vi "Lambda_Configuration4.vi"() -> ()   [LabVIEW 2015]
uses:
  <vilib>/Utility/error.llb/DialogType.ctl
  <vilib>/Platform/TimedLoop/XDataNode/timing_clust.ctl
  <vilib>/Platform/TimedLoop/XDataNode/nitl_modes.ctl
  <vilib>/Platform/TimedLoop/XDataNode/wakeup.ctl
  <vilib>/Utility/file.llb/Read From Spreadsheet File (DBL).vi
  <vilib>/platform/TimedLoop/XDataNode/XDataNode.xnode
  <vilib>/Platform/TimedLoop/XDataNode/XDNodeRunTimeDep.lvlib
panel:
  in  "?":bool
  out "Voltage":dbl[](graph)
  out "Current":dbl[](graph)
  in  "?":bool
  out "Output Current":dbl format="%.4f"
  out "Output Voltage":dbl format="%.4f"
  out "Serial Number:":string
  out "error?":bool
  out "Model:":string
  in  "Reset (T)":bool=TRUE
  in  "BAUD":u16(ring)=3 items=["1200", "2400", "4800", "9600", "19200"]
  in  "GEN Addr":i16=6
  in  "VISA name":refnum<visa-resource-name>
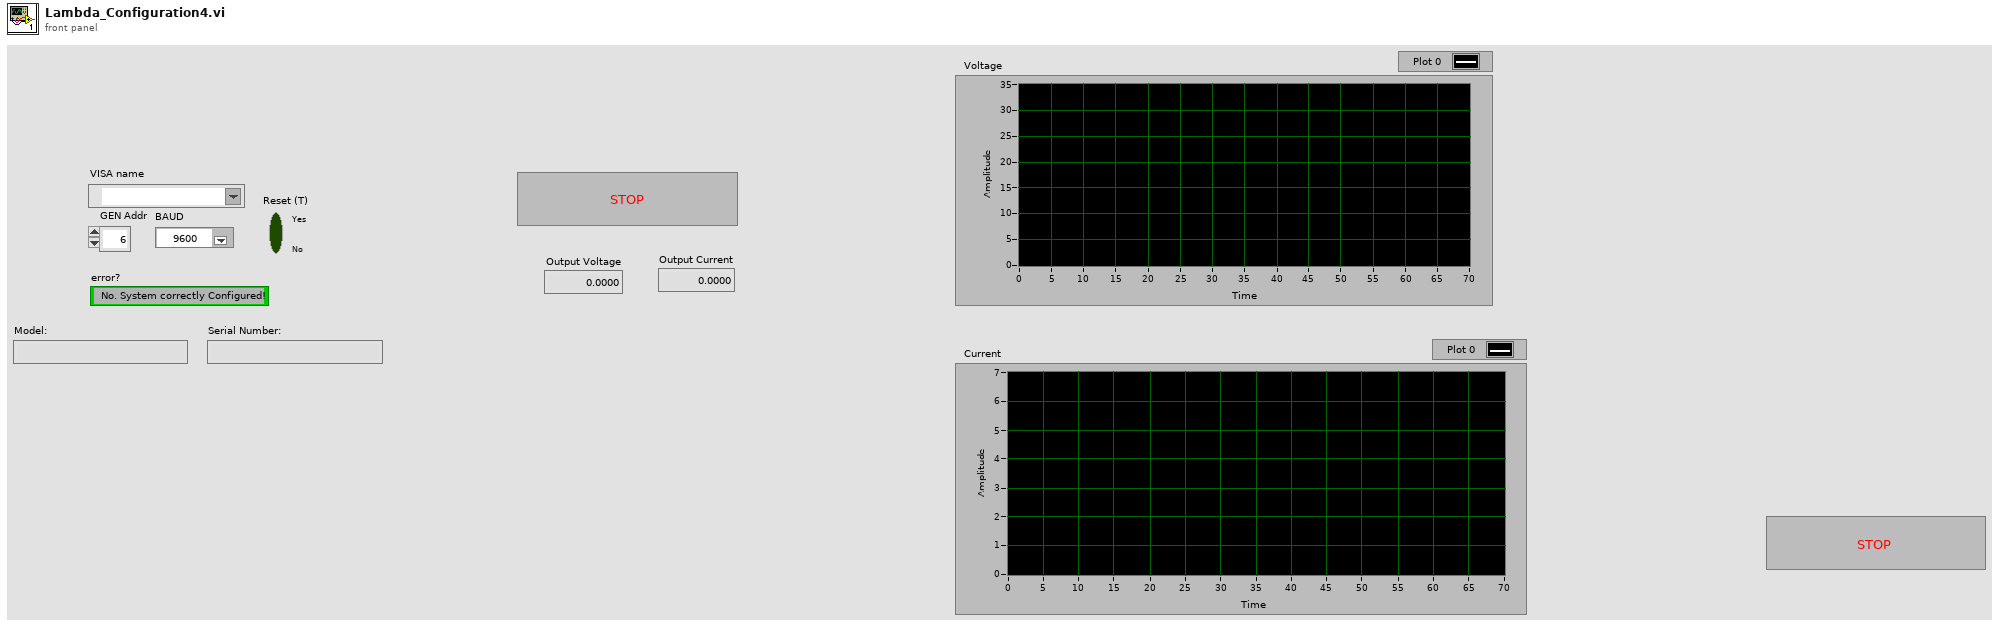
[diagram p1: front panel]
types:
  T1 = typedef "XDNodeRunTimeDep.lvlib/timing_clust.ctl" = cluster{"Expected End [f-1]":u64, "Actual End [f-1]":u64, "Finished Late? [f-1]":bool, "Expected End [i-1]":u64, "Actual End [i-1]":u64, "Finished Late? [i-1]":bool, "Expected Start [i]":u64, "Actual Start [i]":u64, "Expected Start [f]":u64, "Actual Start [f]":u64, "Source Name":string, "Structure Name":string, "Period":i64, "Deadline":i64, "Offset":i64, "Start":i64, "Priority":i32, "Timeout":i32, "Mode":T2, "Wakeup Reason":T3, "Error":errorcluster, "Source Type":string, "Secondary Source Type":string, "Global End Time":u64, "Global Start Time":u64, "Frame Duration":u64, "Iteration Duration":u64, "Assigned CPU":i32, "I/O Scan Engine Mode":u32}
  T2 = typedef "XDNodeRunTimeDep.lvlib/nitl_modes.ctl" = enum32{"No Change", "Process missed periods, maintain original phase", "Discard missed periods, maintain original phase", "Process missed periods, ignore original phase", "Discard missed periods, ignore original phase"}
  T3 = typedef "XDNodeRunTimeDep.lvlib/wakeup.ctl" = enum32{"Normal", "Aborted", "Asynchronous wakeup", "Timing source error", "Timed loop error", "Timeout"}
  T4 = typedef "DialogType.ctl" = u16
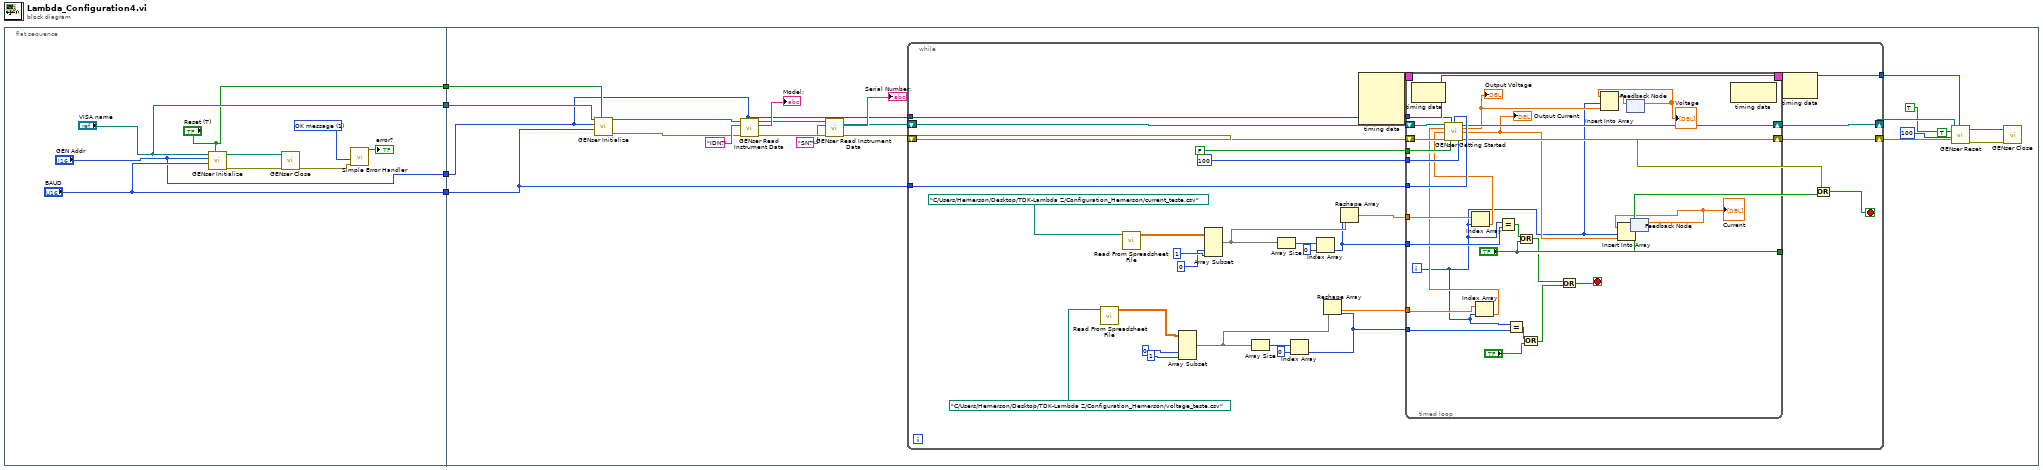
[diagram p0: block diagram]
diagram:
  n1 = flat-sequence {
    tunnel: ["BAUD"] -> w4
    tunnel: ["GEN Addr"] -> w3
    tunnel: ["VISA name"] -> w2
    tunnel: ["Reset (T)"] -> w1
    tunnel: w4 -> [w21]
    tunnel: w3 -> [w22]
    tunnel: w2 -> [w27]
    tunnel: w1 -> [w28]
    frame #0 {
      w10 = T4 1 items=["no dialog", "OK message", "continue or stop message", "OK message + warnings", "continue/stop + warnings"] ("type of dialog (OK msg:1)")
      n2 = call <instrlib>:"GENser Initialize.vi"("Reset (T)"="Reset (T)", "BAUD"="BAUD", "GEN Addr"="GEN Addr", "VISA name"="VISA name") -> ("error out"=w12:errorcluster, "VISA out"=w13:refnum<visa-resource-name>)  [unwired: 6 in]
      n3 = call <instrlib>:"GENser Close.vi"("error"=w12, "VISA name"=w13) -> ("error out"=w11:errorcluster)  [unwired: 9 in]
      n4 = call <vilib>:"Simple Error Handler.vi"("type of dialog (OK msg:1)"=w10, "error in (no error)"=w11) -> ("error?"=→"error?":bool)  [unwired: 3 in, 4 out]
    }
    frame #1 {
      (unwired) TRUE ("Reset (T)")
      n5 = call <instrlib>:"GENser Initialize.vi"("Reset (T)"=w28, "BAUD"=w21, "GEN Addr"=w22, "VISA name"=w27) -> ("error out"=w25:errorcluster, "VISA out"=w26:refnum<visa-resource-name>)  [unwired: 6 in]
      n6 = call <instrlib>:"GENser Read Instrument Data.vi"("GEN Addr"=w22, "error"=w25, "Query"="IDN?", "VISA"=w26) -> ("error out"=w31:errorcluster, "Response"=→"Model:":string, "VISA out"=w32:refnum<visa-resource-name>)  [unwired: 4 in, 1 out]
      n7 = call <instrlib>:"GENser Read Instrument Data.vi"("error"=w31, "Query"="SN?", "VISA"=w32) -> ("error out"=w23:errorcluster, "Response"=→"Serial Number:":string, "VISA out"=w24:refnum<visa-resource-name>)  [unwired: 5 in, 1 out]
      n8 = while {
        tunnel: w22 -> [w57]
        tunnel: w21 -> [w61]
        shift-right: [w58] -> w20
        shift-left: w24 -> [w64]
        shift-right: [w47] -> w19
        shift-left: w23 -> [w62]
        tunnel: [w57] -> w16
        stop <- w60 stop-if-true
        n9 = call-poly <vilib>:"Read From Spreadsheet File.vi"("file path (dialog if empty)"=path "C:/Users/Hemerson/Desktop/TDK-Lambda Z/Configuration_Hemerson/voltage_teste.csv") -> ("all rows"=w35:dbl[][])  [unwired: 6 in, 4 out]
        n10 = call-poly <vilib>:"Read From Spreadsheet File.vi"("file path (dialog if empty)"=path "C:/Users/Hemerson/Desktop/TDK-Lambda Z/Configuration_Hemerson/current_teste.csv") -> ("all rows"=w42:dbl[][])  [unwired: 6 in, 4 out]
        n11 = Array Subset "Array Subset"(array=w35, index (col)=0 ("index"), length (col)=1 ("length")) -> (w39:dbl[][])  [unwired: 2 in]
        n12 = Array Subset "Array Subset"(array=w42, index (col)=0 ("index"), length (col)=1 ("length")) -> (w53:dbl[][])  [unwired: 2 in]
        n13 = Array Size(array=w39) -> (size(s)=w43:i32[])
        n14 = Array Size(array=w53) -> (size(s)=w54:i32[])
        n15 = Index Array "Index Array"(array=w43, index=0) -> (element=w38:i32)
        n16 = Index Array "Index Array"(array=w54, index=0) -> (element=w46:i32)
        n17 = Reshape Array "Reshape Array"(w39, w38) -> (w37:dbl[])
        n18 = Reshape Array "Reshape Array"(w53, w46) -> (w48:dbl[])
        n19 = node-c288() -> (w50:T1)  [unwired: 4 in]
        n20 = timed-loop {
          timing: w50 -> [_]
          timing-out: [_] -> w49
          tunnel: FALSE ("Reset (T)") -> [w91]
          tunnel: w61 -> [w89]
          tunnel: u32 100 ("Settle (0 mS)") -> [w88]
          tunnel: w57 -> [w86]
          shift-right: [w87] -> w58
          shift-left: w64 -> [w92]
          shift-right: [w83] -> w47
          shift-left: w62 -> [w90]
          tunnel: w48 -> [w85]
          tunnel: w46 -> [w81]
          tunnel: ["?"] -> w45
          tunnel: w38 -> [w72]
          tunnel: w37 -> [w71]
          i -> [w66]
          stop <- w65 stop-if-true
          n21 = node-c288() -> ()  [unwired: 1 in, 1 out]
          n22 = Index Array(array=w85, index=w66) -> (element=w84:dbl)
          n23 = Index Array(array=w71, index=w66) -> (element=w67:dbl)
          n24 = call <instrlib>:"GENser Getting Started.vi"("VISA"=w92, "GEN Addr"=w86, "BAUD"=w89, "Voltage Limit"=w67, "Current Limit"=w84, "error"=w90, "Reset (T)"=w91, "Settle (0 mS)"=w88) -> ("VISA out"=w87:refnum<visa-resource-name>, "Output Voltage"=w74:dbl, "Output Current"=w77:dbl, "error out"=w83:errorcluster)  [unwired: 4 in]
          "Output Current" <- w77
          "Output Voltage" <- w74
          n25 = Equal?(x=w66, y=w81) -> (x = y?=w82:bool)
          n26 = Equal?(x=w66, y=w72) -> (x = y?=w70:bool)
          n27 = Or(x=w82, y="?") -> (x .or. y?=w69:bool)
          n28 = Or(x=w70, y="?") -> (x .or. y?=w68:bool)
          n29 = Or(x=w69, y=w68) -> (x .or. y?=w65:bool)
          n30 = feedback #1() -> (w75:dbl[])  [unwired: 1 in]
          "Voltage" <- w75
          n31 = Insert Into Array(array=w75, index=w66, new element=w74) -> (w76:dbl[])
          n32 = feedback-in #1(w76) -> ()
          n33 = feedback #2() -> (w78:dbl[])  [unwired: 1 in]
          "Current" <- w78
          n34 = Insert Into Array(array=w78, index=w66, new element=w77) -> (w79:dbl[])
          n35 = feedback-in #2(w79) -> ()
          n36 = node-c288() -> ()  [unwired: 1 in, 1 out]
        }
        n37 = node-c288(w49) -> ()  [unwired: 1 out]
        n38 = Or(x=w47, y=w45) -> (x .or. y?=w60:bool)
      }
      n39 = call <instrlib>:"GENser Reset.vi"("GEN Addr"=w16, "error"=w19, "Settle (0 mS)"=u32 100, "Reset (T)"=TRUE, "VISA"=w20) -> ("error out"=w14:errorcluster, "VISA out"=w17:refnum<visa-resource-name>)  [unwired: 5 in]
      n40 = call <instrlib>:"GENser Close.vi"("error"=w14, "VISA name"=w17) -> ()  [unwired: 9 in, 1 out]
    }
  }
